vi "Set Param.vi"(8 "error in (no error)":errorcluster, 11 "DelayLineLS4 in":refnum<class "DLLS4.lvclass">) -> (0 "error out":errorcluster, 3 "DelayLineLS4 out":refnum<class "DLLS4.lvclass">)   [LabVIEW 2015, in "DLLS4.lvclass"]
uses:
  DLLS4.lvclass
  LS4 axis.ctl
  DelayLine.lvclass
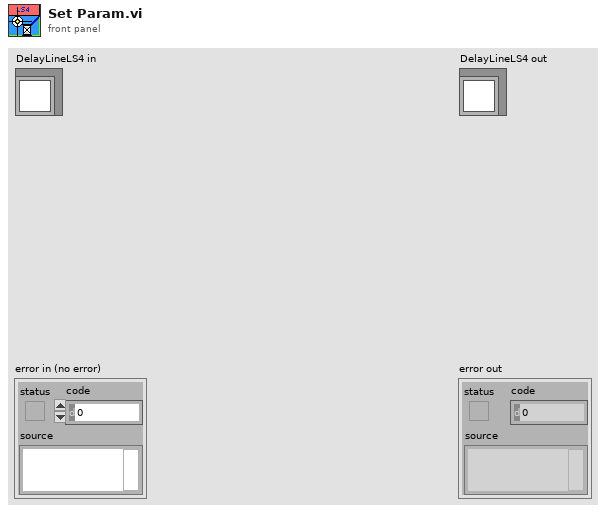
[diagram p1: front panel]
types:
  T1 = typedef "DelayLine.lvclass/LS4 axis.ctl" = u16
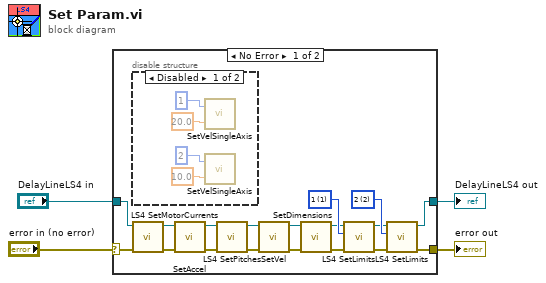
[diagram p0: block diagram]
diagram:
  n1 = case shown="No Error" "error in (no error)" {
    selector: "error in (no error)" -> [w17 w28]
    tunnel: [w7 w28] -> w3
    tunnel: [w8 w27] -> w1
    tunnel: "DelayLineLS4 in" -> [w22 w27]
    frame No Error {
      w11 = T1 2 items=["1"=1, "2"=2, "3"=3, "4"=4] ("Axis")
      w12 = T1 1 items=["1"=1, "2"=2, "3"=3, "4"=4] ("Axis")
      n2 = disable-structure shown="Disabled" {
        frame Disabled {
          n3 = call "SetVelSingleAxis.vi"("Vel"=20.0, "Axis"=1) -> ()  [unwired: 1 out]
          n4 = call "SetVelSingleAxis.vi"("Vel"=10.0, "Axis"=2) -> ()  [unwired: 1 out]
        }
        frame Enabled {
        }
      }
      n5 = call "LS4 SetMotorCurrents.vi"("error in (no error)"=w17, "DelayLineLS4 in"=w22) -> ("error out"=w16:errorcluster, "DelayLineLS4 out"=w21:refnum<class "DLLS4.lvclass">)  [unwired: 8 in]
      n6 = call "SetAccel.vi"("error in (no error)"=w16, "DelayLineLS4 in"=w21) -> ("error out"=w15:errorcluster, "DelayLineLS4 out"=w20:refnum<class "DLLS4.lvclass">)  [unwired: 8 in]
      n7 = call "LS4 SetPitches.vi"("error in (no error)"=w15, "DelayLineLS4 in"=w20) -> ("error out"=w14:errorcluster, "DelayLineLS4 out"=w19:refnum<class "DLLS4.lvclass">)  [unwired: 8 in]
      n8 = call "SetVel.vi"("error in (no error)"=w14, "DelayLineLS4 in"=w19) -> ("error out"=w13:errorcluster, "DelayLineLS4 out"=w18:refnum<class "DLLS4.lvclass">)  [unwired: 8 in]
      n9 = call "SetDimensions.vi"("error in (no error)"=w13, "DelayLineLS4 in"=w18) -> ("error out"=w5:errorcluster, "DelayLineLS4 out"=w10:refnum<class "DLLS4.lvclass">)  [unwired: 8 in]
      n10 = call "LS4 SetLimits.vi"("error in (no error)"=w5, "Axis"=w12, "DelayLineLS4 in"=w10) -> ("error out"=w6:errorcluster, "DelayLineLS4 out"=w9:refnum<class "DLLS4.lvclass">)  [unwired: 7 in]
      n11 = call "LS4 SetLimits.vi"("error in (no error)"=w6, "Axis"=w11, "DelayLineLS4 in"=w9) -> ("error out"=w7:errorcluster, "DelayLineLS4 out"=w8:refnum<class "DLLS4.lvclass">)  [unwired: 7 in]
    }
    frame Error {
    }
  }
  "error out" <- w3
  "DelayLineLS4 out" <- w1
